vi "Read Index.vi"(8 "error in (no error)":errorcluster, 11 "Abs_Type in":refnum<class "Abs_Type.lvclass">) -> (0 "error out":errorcluster, 2 "Index":i32, 3 "Abs_Type out":refnum<class "Abs_Type.lvclass">)   [LabVIEW 2021, in "Abs_Type.lvclass"]
uses:
  Abs_Type.lvclass
  Abs_Type.lvclass/Abs_Type.ctl
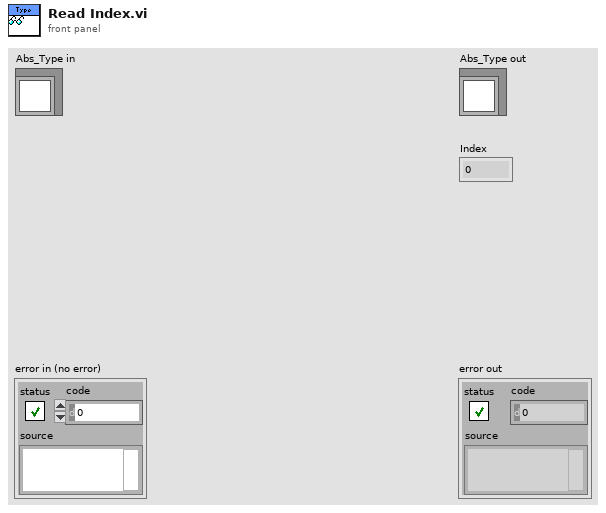
[diagram p1: front panel]
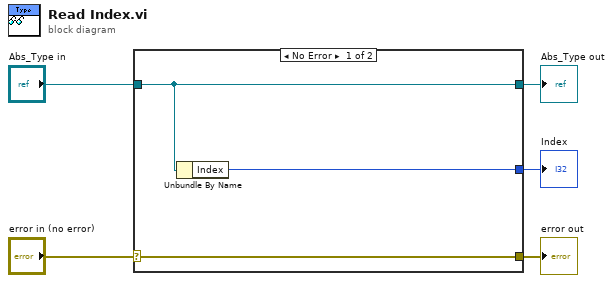
[diagram p0: block diagram]
diagram:
  n1 = case shown="No Error" "error in (no error)" {
    selector: "error in (no error)" -> [w8 w9]
    tunnel: [w8 w9] -> w4
    tunnel: [w7 w10] -> w2
    tunnel: "Abs_Type in" -> [w7 w10]
    tunnel: [w6 _] -> w1
    frame No Error {
      n2 = Unbundle By Name(w7) -> ("Index"=w6:i32)
    }
    frame Error {
    }
  }
  "error out" <- w4
  "Abs_Type out" <- w2
  "Index" <- w1
